vi "Periodic Tasks.vi"(8 "error in":errorcluster) -> ()   [LabVIEW 2018]
doc: "This VI runs in parallel to other robot code. It can contain as many user-defined periodic loops as you need. These can carry out PID or other sorts of timed response."
uses:
  <vilib>/Rock Robotics/WPI/Utilities/WPI_GetSetVariantRefNum.vi
panel:
  out "Waveform Chart 3":T1(graph)
  out "Waveform Chart 2":T2(graph)
  out "Waveform Chart":dbl(graph)
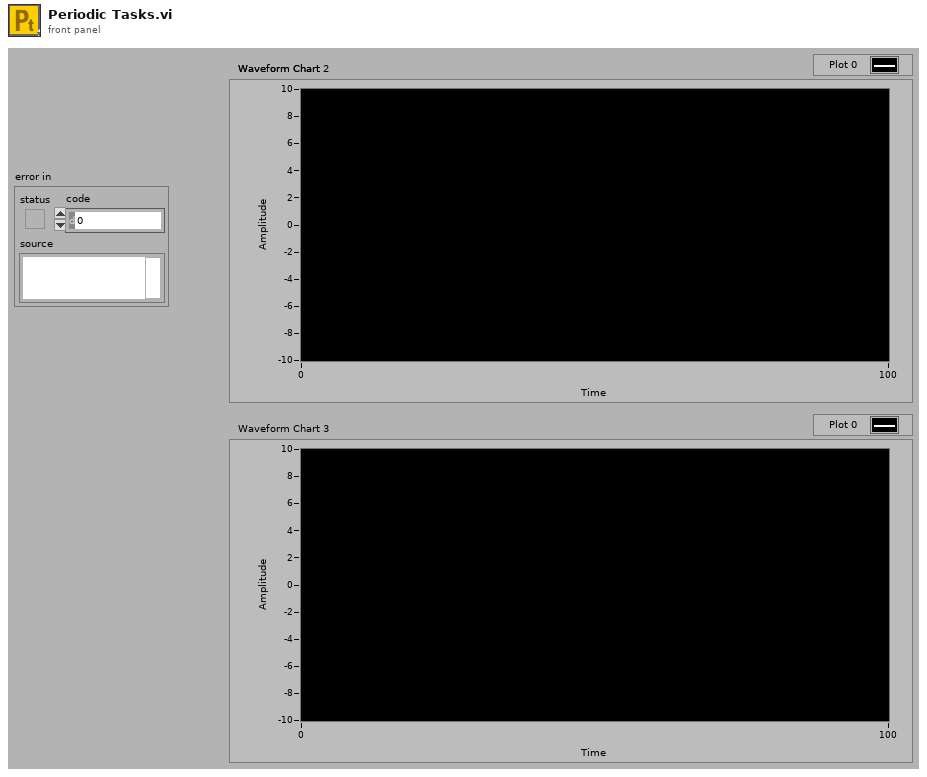
[diagram p1: front panel]
types:
  T1 = cluster{"Sensor Velocity":dbl, "Sensor Velocity":dbl, "Sensor Velocity":dbl}
  T2 = cluster{"Motor Temperature":u8, "Motor Temperature":u8, "Motor Temperature":u8}
  T3 = typedef "WPI_JoystickDevRef.ctl" = cluster{"Device":T4}
  T4 = typedef "WPI_JoystickDeviceEnum.ctl" = enum16{"USB 0", "USB 1", "USB 2", "USB 3", "USB 4", "USB 5"}
  T5 = typedef "SPARKMAX6Motor.ctl" = cluster{"FrontLeftMaster":T6, "FrontLeftSlave1":T6, "FrontLeftSlave2":T6, "FrontRightMaster":T6, "FrontRightSlave1":T6, "FrontRightSlave2":T6}
  T6 = typedef "WPI_MotorControlDeviceRef.ctl" = cluster{"DeviceStatus":errorcluster, "Type":T7, "PWM":cluster{"PWM Channel":T8, "DeadBand":T9}, "CAN":cluster{"Device Number":u8, "SetOutput VI Ref":variant, "GetOutput VI Ref":variant, "Enable VI Ref":variant, "Disable VI Ref":variant, "Data":variant}, "Invert":bool, "DIO PWM":cluster{"PWM \"Enable\" Channel":T8, "DIOChannel":T10, "PWM Rate":dbl}}
  T7 = typedef "WPI_MotorControlType.ctl" = enum16{"PWM", "CAN", "DIO PWM"}
  T8 = typedef "FPGA_DIOPWMChannel.ctl" = enum8{"PWM 0", "PWM 1", "PWM 2", "PWM 3", "PWM 4", "PWM 5", "PWM 6", "PWM 7", "PWM 8", "PWM 9", "PWM MXP 0", "PWM MXP 1", "PWM MXP 2", "PWM MXP 3", "PWM MXP 4", "PWM MXP 5", "PWM MXP 6", "PWM MXP 7", "PWM MXP 8", "PWM MXP 9", "Invalid"}
  T9 = typedef "WPI_PWMDeadband.ctl" = cluster{"Name":string, "maxPositivePwm":i32, "minPositivePwm":i32, "centerPwm":i32, "maxNegativePwm":i32, "minNegativePwm":i32, "angularRange":u16}
  T10 = typedef "FPGA_DIOChannel.ctl" = enum8{"DIO 0", "DIO 1", "DIO 2", "DIO 3", "DIO 4", "DIO 5", "DIO 6", "DIO 7", "DIO 8", "DIO 9", "DIO MXP 0", "DIO MXP 1", "DIO MXP 2", "DIO MXP 3", "DIO MXP 4", "DIO MXP 5", "DIO MXP 6", "DIO MXP 7", "DIO MXP 8", "DIO MXP 9", "DIO MXP 10", "DIO MXP 11", "DIO MXP 12", "DIO MXP 13", "DIO MXP 14", "DIO MXP 15", "SPI Port CS1", "SPI Port CS2", "SPI Port CS3", "SPI Port MISO", "SPI Port MOSI", "Invalid"}
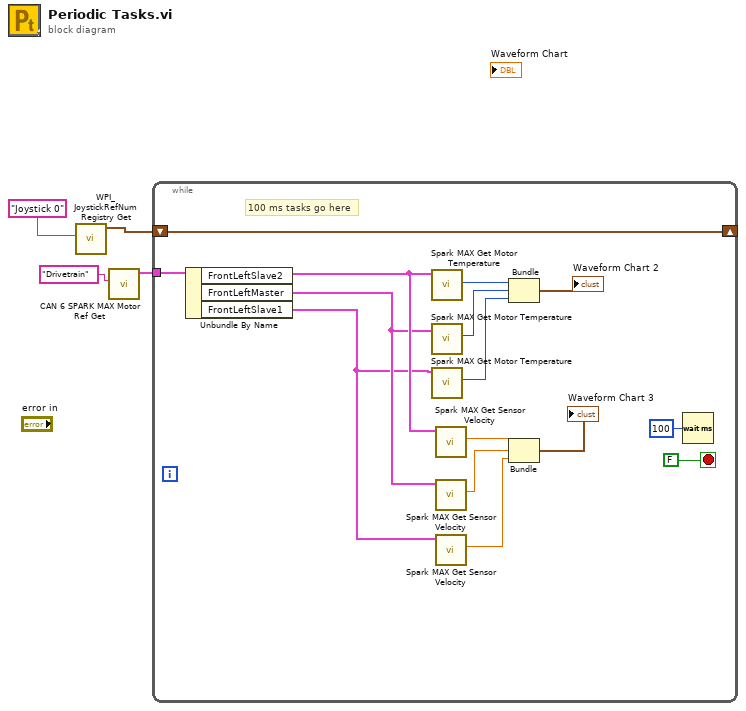
[diagram p0: block diagram]
diagram:
  n1 = call <vilib>:"WPI_JoystickRefNum Registry Get.vi"("refnum name"="Joystick 0") -> ("JoystickDevRef"=w3:T3)  [unwired: 1 in, 9 out]
  n2 = call "CAN 6 SPARK MAX Motor Ref Get.vi"("refnum name"="Drivetrain") -> ("TalonSRX6MotorRef out"=w1:T5)  [unwired: 9 in, 1 out]
  n3 = while {
    shift-right: [w17] -> _
    shift-left: w3 -> [w17]
    tunnel: w1 -> [w16]
    stop <- FALSE stop-if-true
    # "100 ms tasks go here"
    n4 = Unbundle By Name(w16) -> ("FrontLeftSlave2"=w7:T6, "FrontLeftMaster"=w6:T6, "FrontLeftSlave1"=w5:T6)
    n5 = call <vilib>:"Spark MAX Get Motor Temperature.vi"("MotorControlDevRef in"=w7) -> ("Motor Temperature"=w15:u8)  [unwired: 7 in, 3 out]
    n6 = call <vilib>:"Spark MAX Get Motor Temperature.vi"("MotorControlDevRef in"=w6) -> ("Motor Temperature"=w14:u8)  [unwired: 7 in, 3 out]
    n7 = call <vilib>:"Spark MAX Get Motor Temperature.vi"("MotorControlDevRef in"=w5) -> ("Motor Temperature"=w13:u8)  [unwired: 7 in, 3 out]
    n8 = call <vilib>:"Spark MAX Get Sensor Velocity.vi"("MotorControlDevRef in"=w7) -> ("Sensor Velocity"=w11:dbl)  [unwired: 7 in, 3 out]
    n9 = call <vilib>:"Spark MAX Get Sensor Velocity.vi"("MotorControlDevRef in"=w6) -> ("Sensor Velocity"=w10:dbl)  [unwired: 7 in, 3 out]
    n10 = call <vilib>:"Spark MAX Get Sensor Velocity.vi"("MotorControlDevRef in"=w5) -> ("Sensor Velocity"=w9:dbl)  [unwired: 7 in, 3 out]
    n11 = Bundle("Motor Temperature"=w15, "Motor Temperature"=w14, "Motor Temperature"=w13) -> (→"Waveform Chart 2":T2)  [unwired: 1 in]
    n12 = Bundle("Sensor Velocity"=w11, "Sensor Velocity"=w10, "Sensor Velocity"=w9) -> (→"Waveform Chart 3":T1)  [unwired: 1 in]
    n13 = Wait (ms)(milliseconds to wait=u32 100) -> ()  [unwired: 1 out]
  }
